vi "Idle Exit Action.vi"(8 "error in (no error)":errorcluster caption="错误输入（无错误）", 9 "Exit Action":bool, 11 "SM Data In":T1) -> (0 "error out":errorcluster caption="错误输出", 3 "SM Data Out":T1)   [LabVIEW 2013, in "标准状态机模板.lvlib"]
uses:
  Control/SM Data.ctl
  Control/State.ctl
  Control/Input Data.ctl
  Control/Output Data.ctl
  Control/Internal Data.ctl
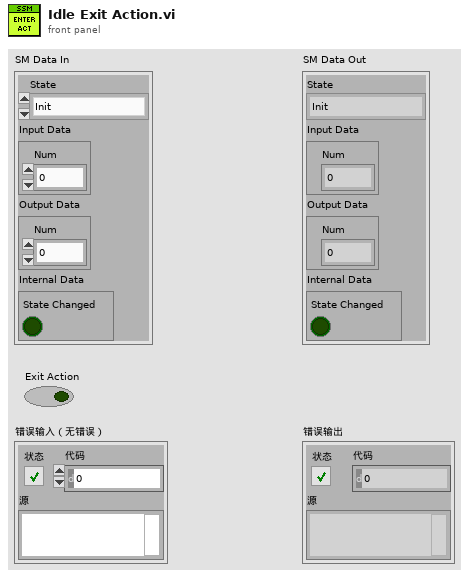
[diagram p1: front panel]
types:
  T1 = typedef "标准状态机模板.lvlib/SM Data.ctl" = cluster{"State":T2, "Input Data":T3, "Output Data":T4, "Internal Data":T5}
  T2 = typedef "标准状态机模板.lvlib/State.ctl" = enum16{"Init", "Idle"}
  T3 = typedef "标准状态机模板.lvlib/Input Data.ctl" = cluster{"Num":dbl}
  T4 = typedef "标准状态机模板.lvlib/Output Data.ctl" = cluster{"Num":dbl}
  T5 = typedef "标准状态机模板.lvlib/Internal Data.ctl" = cluster{"State Changed":bool}
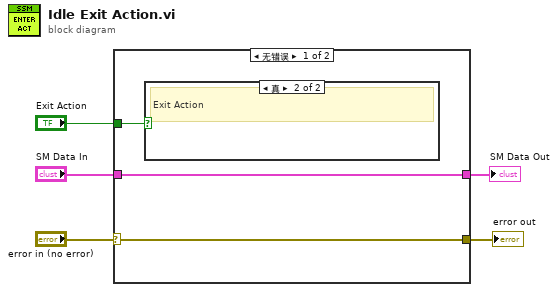
[diagram p0: block diagram]
diagram:
  n1 = case shown="无错误" "error in (no error)" {
    selector: "error in (no error)" -> [w7 w9]
    tunnel: "SM Data In" -> [w8 w10]
    tunnel: [w8 w10] -> w3
    tunnel: [w7 w9] -> w2
    tunnel: "Exit Action" -> [w6 _]
    frame No Error {
      n2 = case shown="真" w6 {
        frame False {
        }
        frame True {
          # "Exit Action"
        }
      }
    }
    frame Error {
    }
  }
  "error out" <- w2
  "SM Data Out" <- w3
